vi "Select top data.vi"(7 "condition":string, 8 "error in (no error)":errorcluster, 9 "Row":i32, 10 "table":string, 11 "connection reference":T1) -> (0 "error out":errorcluster, 2 "recordset data":variant[][](array[variant]), 3 "connection reference out":T1)   [LabVIEW 2014]
uses:
  <vilib>/addons/database/NI_Database_API.lvlib
  <vilib>/addons/database/Recordset.llb/Rec Destroy - Connection.vi
  <vilib>/addons/database/Connection.llb/Conn Execute.vi
  <vilib>/addons/database/Recordset.llb/Rec Fetch Recordset Data (R).vi
  <vilib>/addons/database/Connection.llb/Conn ObjectReference.ctl
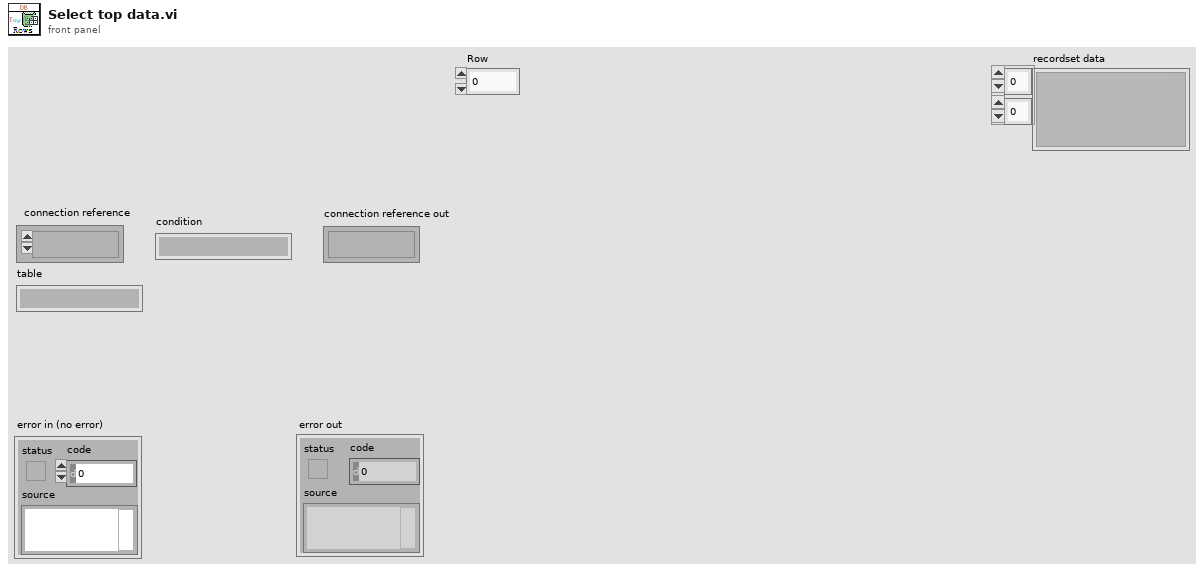
[diagram p1: front panel]
types:
  T1 = typedef "NI_Database_API.lvlib/Conn ObjectReference.ctl" = refnum<k1>
  T2 = typedef "NI_Database_API.lvlib/Rec ObjectReference.ctl" = refnum<k1>
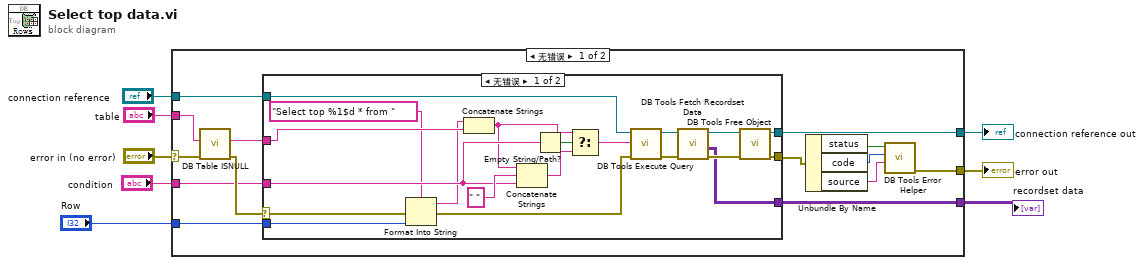
[diagram p0: block diagram]
diagram:
  n1 = case shown="无错误" "error in (no error)" {
    selector: "error in (no error)" -> [w11 w46]
    tunnel: "table" -> [w22 _]
    tunnel: [w15 w46] -> w7
    tunnel: [w14 w45] -> w6
    tunnel: "connection reference" -> [w13 w45]
    tunnel: "condition" -> [w12 _]
    tunnel: [w10 _] -> w2
    tunnel: "Row" -> [w9 _]
    frame No Error {
      n2 = call "DB Table ISNULL.vi"("error in (no error)"=w11, "table"=w22) -> ("error out"=w19:errorcluster, "table out"=w20:string)  [unwired: 8 in]
      n3 = case shown="无错误" w19 {
        selector: w19 -> [w27 w44]
        tunnel: w20 -> [w31 _]
        tunnel: [w42 w44] -> w21
        tunnel: [w34 w43] -> w14
        tunnel: w13 -> [w32 w43]
        tunnel: w12 -> [w33 _]
        tunnel: [w28 _] -> w10
        tunnel: w9 -> [w24 _]
        frame No Error {
          n4 = Format Into String(format string="Select top %1$d * from ", error in=w27, w24) -> (resulting string=w23:string, error out=w26:errorcluster)  [unwired: 1 in]
          n5 = Concatenate Strings(w23, w31) -> (w30:string)
          n6 = Concatenate Strings(w30, " " ("Substring"), w33) -> (w37:string)
          n7 = Empty String/Path?(string/path=w33) -> (empty?=w38:bool)
          n8 = Select(t=w30, s=w38, f=w37) -> (s? t:f=w35:string)
          n9 = call-poly <vilib>:"DB Tools Execute Query.vi"("error in (no error)"=w26, "SQL query"=w35, "connection reference"=w32) -> ("error out"=w39:errorcluster, "recordset reference"=w40:T2)  [unwired: 5 in]
          n10 = call-poly <vilib>:"DB Tools Fetch Recordset Data.vi"("error in (no error)"=w39, "recordset reference"=w40) -> ("error out"=w29:errorcluster, "recordset data"=w28:variant[][], "recordset reference out"=w41:T2)  [unwired: 3 in]
          n11 = call-poly <vilib>:"DB Tools Free Object.vi"("error in (no error)"=w29, "recordset reference"=w41) -> ("error out"=w42:errorcluster, "connection reference"=w34:T1)  [unwired: 8 in]
        }
        frame Error {
        }
      }
      n12 = Unbundle By Name(w21) -> ("status"=w18:bool, "code"=w17:i32, "source"=w16:string)
      n13 = call <vilib>:"DB Tools Error Helper.vi"("source"=w16, "code"=w17, "status"=w18) -> ("error out"=w15:errorcluster)  [unwired: 8 in]
    }
    frame Error {
    }
  }
  "error out" <- w7
  "connection reference out" <- w6
  "recordset data" <- w2
